vi "Write Number.vi"(8 "error in (no error)":errorcluster, 10 "Number":dbl, 11 "Number in":refnum<class "Number.lvclass">) -> (0 "error out":errorcluster, 3 "Number out":refnum<class "Number.lvclass">)   [LabVIEW 2023, in "Number.lvclass"]
uses:
  Number.lvclass
  Number.lvclass/Number.ctl
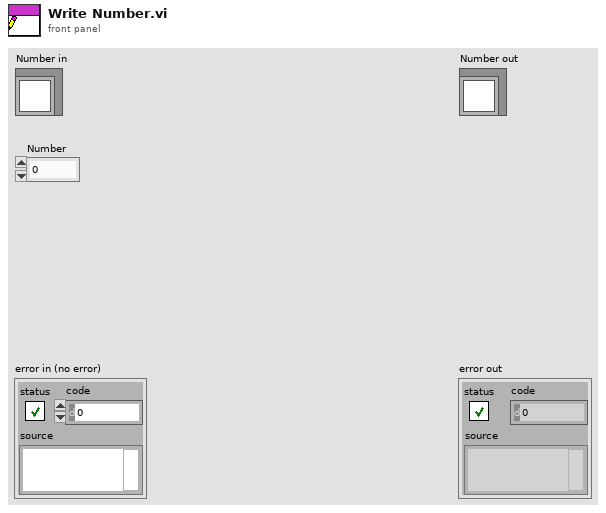
[diagram p1: front panel]
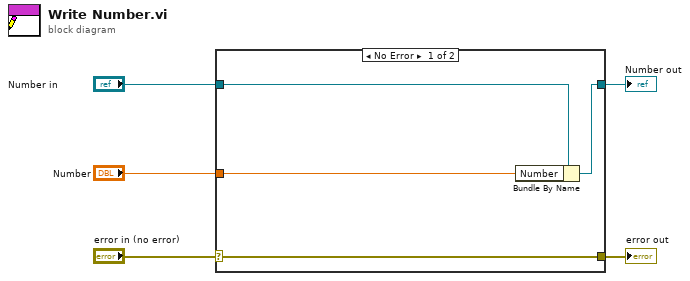
[diagram p0: block diagram]
diagram:
  n1 = case shown="No Error" "error in (no error)" {
    selector: "error in (no error)" -> [w9 w10]
    tunnel: [w9 w10] -> w4
    tunnel: [w7 w11] -> w2
    tunnel: "Number in" -> [w8 w11]
    tunnel: "Number" -> [w6 _]
    frame No Error {
      n2 = Bundle By Name(cluster=w8, "Number"=w6) -> (w7:refnum<class "Number.lvclass">)
    }
    frame Error {
    }
  }
  "error out" <- w4
  "Number out" <- w2
